vi "AssembleBLMultiplotScript-UandTI-CPPPNG.vi"(0 "name or relative path":string, 1 "Final Title":string, 2 "Spectra?":bool, 3 "NormaliseHeight?":bool, 4 "Zref":dbl, 5 "Fit Zmax":dbl, 6 "Fit Zmin":dbl, 7 "HeightJitter%":dbl, 8 "Scale":dbl, 9 "BL Targets":T2[](array[typedef]) {"n" min=0.02 max=0.5 step=0.01 format="%.2f"}, 10 "U,L(U)":refnum<vi>, 11 "UtargetsInfo":T1(array[cluster]), 12 "TI,Sigma":refnum<vi>, 13 "TItargetsInfo":T1(array[cluster]), 15 "No d0":cluster{"n":dbl, "d0":dbl, "d0 2":dbl}, 17 "with d0":cluster{"n":dbl, "d0":dbl, "d0 2":dbl}) -> (20 "gnuplotOut":string)   [LabVIEW 2015]
uses:
  BLTarget.ctl
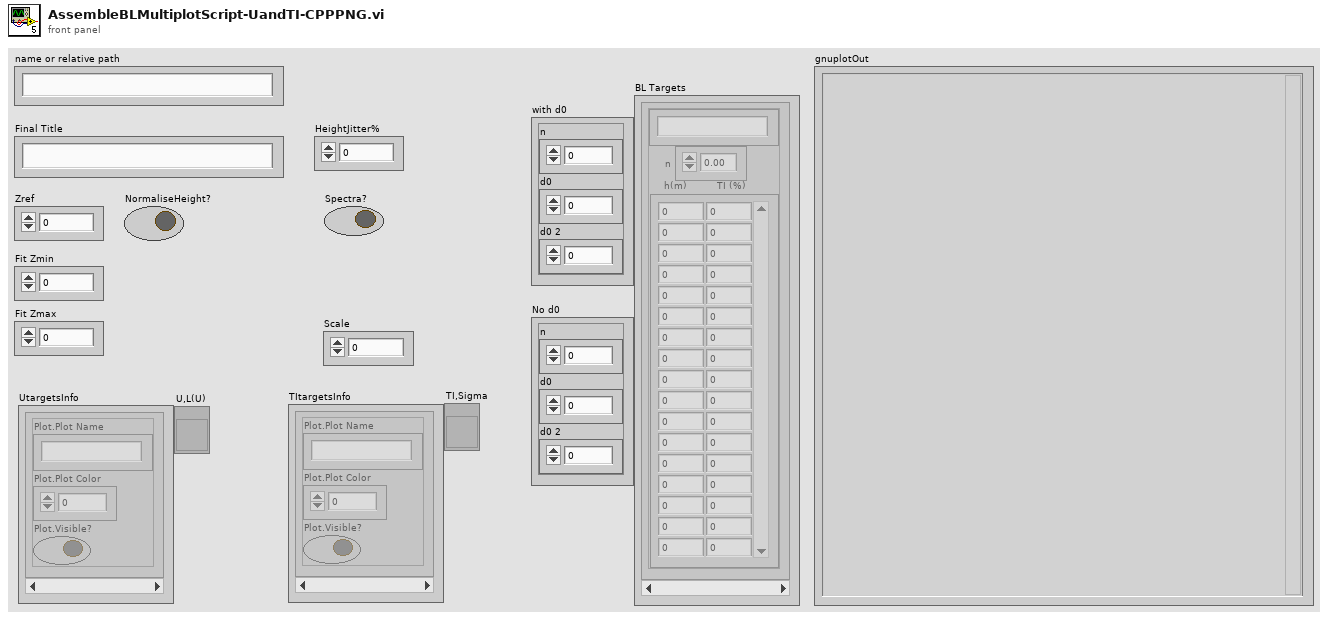
[diagram p1: front panel]
types:
  T1 = cluster{"Plot.Plot Name":string, "Plot.Plot Color":u32, "Plot.Visible?":bool}[]
  T2 = typedef "BLTarget.ctl" = cluster{"Code":string, "TI Profile (FS)":dbl[][], "n":dbl}
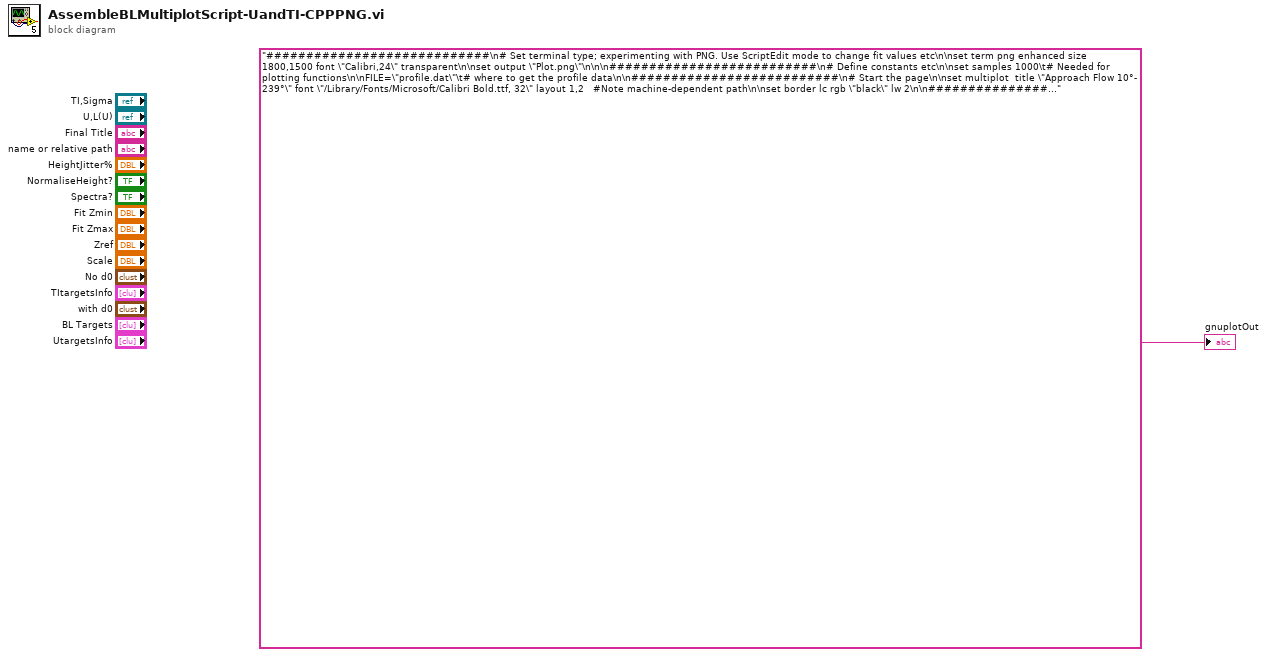
[diagram p0: block diagram]
diagram:
  "gnuplotOut" <- "############################\n# Set terminal type; experimenting with PNG. Use ScriptEdit mode to change fit values etc\n\nset term png enhanced size 1800,1500 font \"Calibri,24\" transparent\n\nset output \"Plot.png\"\n\n\n##########################\n# Define constants etc\n\nset samples 1000\t# Needed for plotting functions\n\nFILE=\"profile.dat\"\t# where to get the profile data\n\n##########################\n# Start the page\n\nset multiplot  title \"Approach Flow 10°- 239°\" font \"/Library/Fonts/Microsoft/Calibri Bold.ttf, 32\" layout 1,2   #Note machine-dependent path\n\nset border lc rgb \"black\" lw 2\n\n############################\n# Margin size per plot, in characters\n\nset tmargin 1.5\nset bmargin 4\nset lmargin 4\nset rmargin 4\n\n############################\n# Fit Equations\n\npowerlaw(U)=zref*U**(1/n)+d  # define inverse power law equation- since the plot is transposed\nclippedpowerlaw(U)=(powerlaw(U)>fitmin && powerlaw(U)<fitmax) ? powerlaw(U) : 1/0 # clip over desired z range\n\n\n############################\n# Plot legend (key) setup\n\nset key samplen 0.9 at first 0, 1.3 left center \n\n\n############################\n# y  axis setup\n\nunset logscale y\nset yrange [0.000000:1.400]\nset mytics 2\nset grid ytics nomytics ls 1 lc rgb \"gray25\"\nunset yzeroaxis\nset ytics 0,0.2,1.4 in mirror format ''\n\nset label center at screen 0.5, first 0.925 \"Height\\n Z/Z_{ref}\"\n\n\n############################\n# TopLeft\n\n#set title \"Mean Profile\"\n\nset label  \"Z_{ref}\" at first 0.07,0.995\nset label  font \",18\" \"full scale:\" at first 0.45,1.015 right\nset label  font \",18\" \" 1312.5ft\" at first 0.45,1.015 left\nset label  font \",18\" \"model scale:\" at first 0.45,0.975 right\nset label  font \",18\" \" 31.5in\" at first 0.45,0.975 left\n\n############################\n# axis setup\n\nset y2label  \"   \" #to balance the Y-numbers on the TI graph\n\n\nunset logscale x\nset xlabel 'Mean Velocity, U/U_{ref}'\nset xrange [0.000000:1.400000]\nset format x\nset xtics autofreq out nomirror \nset mxtics 2\nset grid xtics nomxtics ls 1 lc rgb \"gray25\"\nunset xzeroaxis\nset xtics format '%g'\n\n\n############################\n# Velocity and lengthscale graph\n\n\nplot \\\nfitmin = 0.15, fitmax=1.6, zref=1, d=0, n=0.22, clippedpowerlaw(x) w line ls 1 lw 3 lc rgb \"black\" title 'Power Law, n=0.22', \\\nFILE index 0 using 1:2 axes x1y1 title '' w points lc rgb \"#000080\" pt 6 ps 2.5\n\n\n\n############################\n# TopRight\n\n#set title \"Turbulence Profile\"\n\n\n############################\n# Turn off labels from previous graph\n\nunset label\n\n############################\n# axis setup\n\nunset ylabel\nunset y2label\nset ytics format '%.1f' offset -1.8 # Central Y-scale numbers\n\n\nunset logscale x\nset xlabel \"Turbulence Intensity, u'/U (%)\"\nset xrange [0.0:30.0]\nset format x\nset xtics autofreq out nomirror \nset mxtics 2\n#set grid xtics nomxtics ls 1 lc rgb \"gray25\"\nunset xzeroaxis\nset xtics format '%g'\nset grid xtics nox2tics nomx2tics ls 1 lc rgb \"gray25\"\n\n\n############################\n# TI and sigma graph\n\nplot \\\nFILE index 2 using 1:2 axes x1y1 title '' w points lc rgb '#000080' pt 6 ps 2.5\n\n#Multiplot still needs closing out, but that's handled by a later case...\n"
